vi "Send Receive Parse.vi"(0 "<JSON>":string, 5 "error in (no error)":errorcluster) -> (14 "results-JSON string":string, 19 "error out":errorcluster)   [LabVIEW 2023, in "GenericDevice.lvclass"]
uses:
  GenericDevice.lvclass
  GenericDevice.lvclass/GenericDevice.ctl
  Libraries/DeviceManager/DeviceManager.lvlib
  Communicator/Communicator.lvclass
panel:
  out "error string (if existing)":string
  out "returned command":string
  out "ID":i32
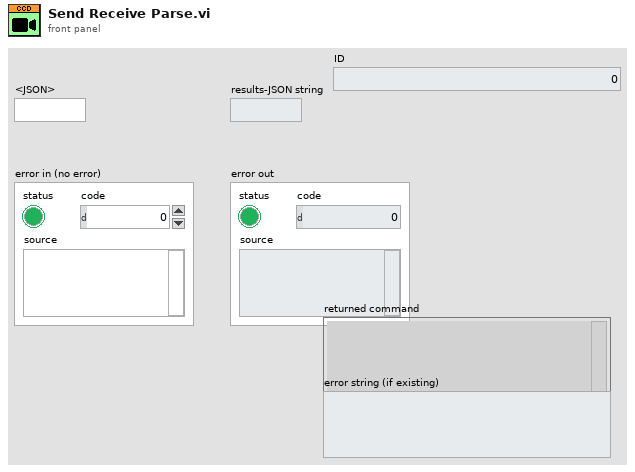
[diagram p1: front panel]
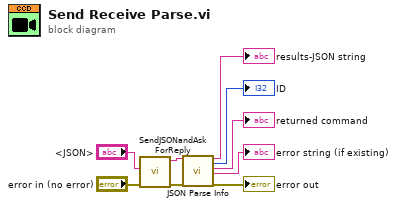
[diagram p0: block diagram]
diagram:
  n1 = call "SendJSONandAskForReply.vi"("error in"="error in (no error)", "JSON to be sent"="<JSON>") -> ("error out"=w6:errorcluster, "JSON reply"=w7:string)  [unwired: 7 in, 1 out]
  n2 = call "JSON Parse Info.vi"("JSON"=w7, "error in (no error)"=w6) -> ("results-JSON"=→"results-JSON string":string, "ID"=→"ID":i32, "returned command"=→"returned command":string, "error string (if existing)"=→"error string (if existing)":string, "error out"=→"error out":errorcluster)  [unwired: 9 in, 4 out]
